vi "Create Trigger Model ConfigList Prev Index Block.vi"(8 "error in (no error)":errorcluster, 9 "Configuration List Name":string="SOURCE_LIST", 10 "Block Number (1)":i32=1 min=1 format="%#.6g", 11 "VISA resource name":refnum<visa-resource-name>) -> (0 "error out":errorcluster, 3 "VISA resource name out":refnum<visa-resource-name>)   [LabVIEW 2021, in "Keithley DMM7510.lvlib"]
doc: "This vi defines a trigger model block that recalls the settings stored at the previous index point in a configuration list."
uses:
  Keithley DMM7510.lvlib
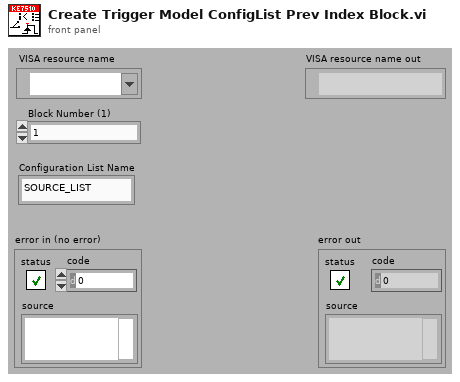
[diagram p1: front panel]
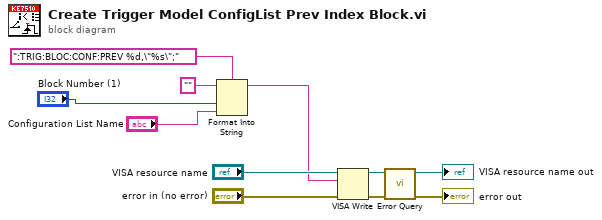
[diagram p0: block diagram]
diagram:
  n1 = Format Into String(format string=":TRIG:BLOC:CONF:PREV %d,\"%s\";", initial string="", "Block Number (1)", "Configuration List Name") -> (resulting string=w2:string)  [unwired: 1 in, 1 out]
  n2 = VISA Write(VISA resource name="VISA resource name", write buffer=w2, error in (no error)="error in (no error)") -> (VISA resource name out=w7:refnum<visa-resource-name>, error out=w6:errorcluster)  [unwired: 1 out]
  n3 = call "Error Query.vi"("error in (no error)"=w6, "VISA resource name"=w7) -> ("error out"=→"error out":errorcluster, "VISA resource name out"=→"VISA resource name out":refnum<visa-resource-name>)  [unwired: 8 out]
